vi "Error Index.vi"() -> ()   [LabVIEW 2015]
panel:
  in  "Error Index":enum16{"0", "1", "2"}(ring)
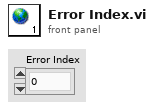
[diagram p1: front panel]
diagram:
